vi "Sandbox calc t0 a.vi"() -> ()   [LabVIEW 2019]
uses:
  TypeDef/Setting Pressure PI.ctl
panel:
  out "A 2":dbl
  in  "milliseconds to wait":u32=10
  out "Waveform Chart":dbl(graph)
  out "x*y":dbl
  in  "Pump":T1={"P [MPa]"=0.0, "A [MPa/V]"=0.0, "P0 [MPa]"=0.0, "P start [%]"=4.0, "P end [%]"=3.5, "T0 DUT [s]"=0.0, "T0 CMBR [s]"=0.0} {"P end [%]" format="%#_13g"; "P start [%]" format="%#_13g"}
  out "#n":dbl
  in  "Time":i32=1000
  out "Waveform Graph":dbl[](graph)
  out "T0":dbl
  in  "T0 in":dbl
  in  "A":dbl
  in  "U":dbl
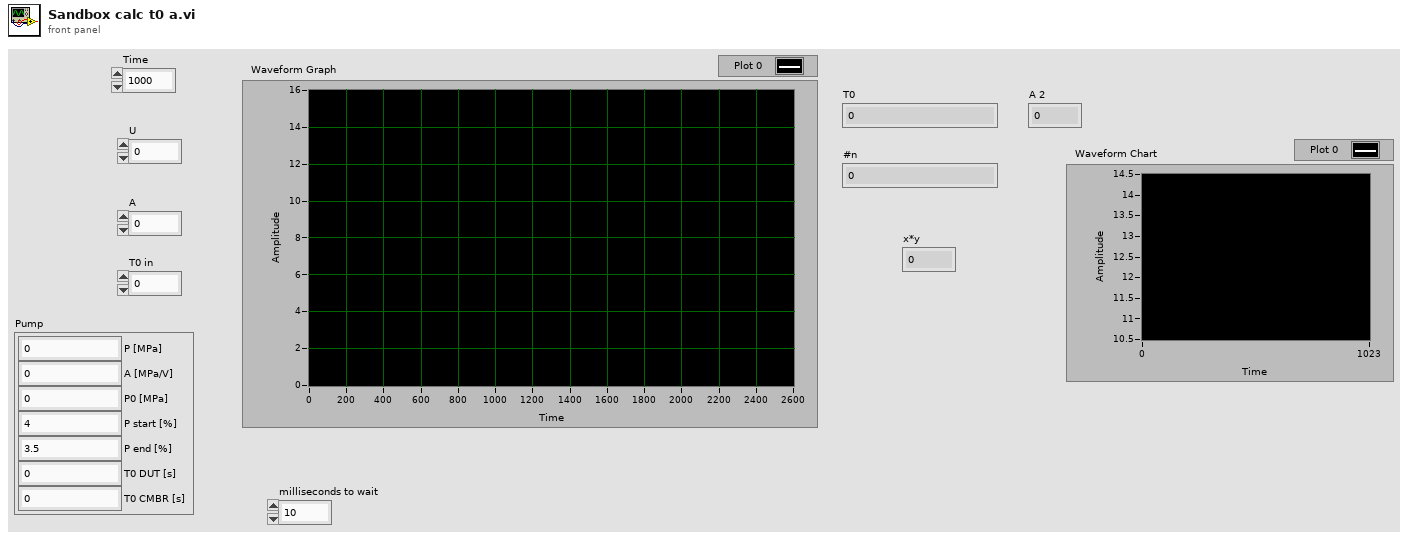
[diagram p1: front panel]
types:
  T1 = typedef "Setting Pressure PI.ctl" = cluster{"P [MPa]":dbl, "A [MPa/V]":dbl, "P0 [MPa]":dbl, "P start [%]":dbl, "P end [%]":dbl, "T0 DUT [s]":dbl, "T0 CMBR [s]":dbl}
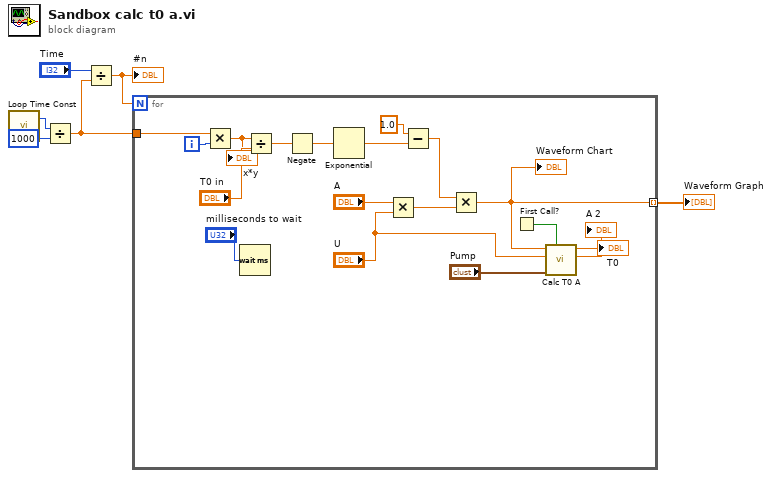
[diagram p0: block diagram]
diagram:
  n1 = call "Loop Time Const.vi"() -> ("loop time ms"=w4:i64)  [unwired: 3 in]
  n2 = Divide(x=w4, y=i64 1000) -> (x/y=w1:dbl)
  n3 = Divide(x="Time", y=w1) -> (x/y=w3:dbl)
  "#n" <- w3
  n4 = for {
    N: w3 -> [_]
    tunnel: [w8] -> w6 mode=indexing
    tunnel: w1 -> [w15]
    i -> [w23]
    n5 = Multiply(x=w15, y=w23) -> (x*y=w13:dbl)
    "x*y" <- w13
    n6 = Wait (ms)(milliseconds to wait="milliseconds to wait") -> ()  [unwired: 1 out]
    n7 = Divide(x=w13, y="T0 in") -> (x/y=w21:dbl)
    n8 = Negate(x=w21) -> (-x=w12:dbl)
    n9 = Exponential(1:w12) -> (0:w11:dbl)
    n10 = Multiply(x="A", y="U") -> (x*y=w18:dbl)
    n11 = Subtract(x=1.0, y=w11) -> (x-y=w10:dbl)
    n12 = Multiply(x=w10, y=w18) -> (x*y=w8:dbl)
    "Waveform Chart" <- w8
    n13 = First Call?() -> (First Call?: T/F=w24:bool)
    n14 = call "Calc T0 A.vi"("init"=w24, "Pump"="Pump", "U"="U", "P"=w8) -> ("A"=→"A 2":dbl, "T0"=→"T0":dbl)  [unwired: 5 in, 1 out]
  }
  "Waveform Graph" <- w6
